vi "CreateArrayHeadersFromRoutineEntries.vi"(0 "Available Routines":string[][](table), 5 "error in":errorcluster) -> (14 "Available Routines out":string[][](table), 15 "Column Headers":string[](array[string]), 16 "Row Headers":string[](array[string]), 19 "error out":errorcluster)   [LabVIEW 2014]
doc: "This VI creates the array headers for the fast alignment routine managing VIs."
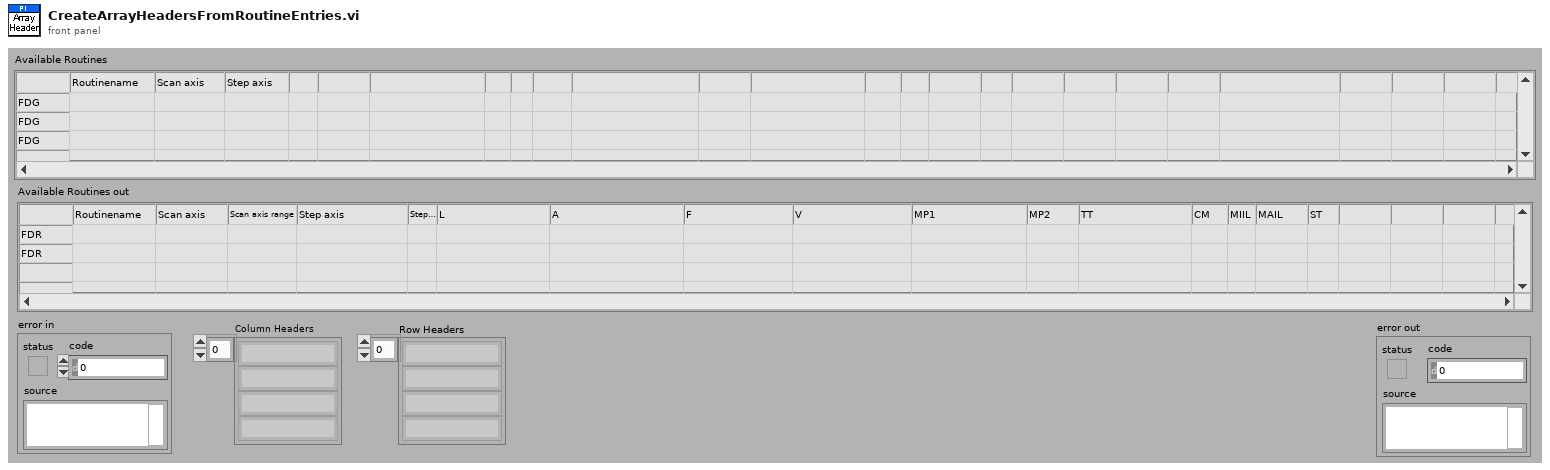
[diagram p1: front panel]
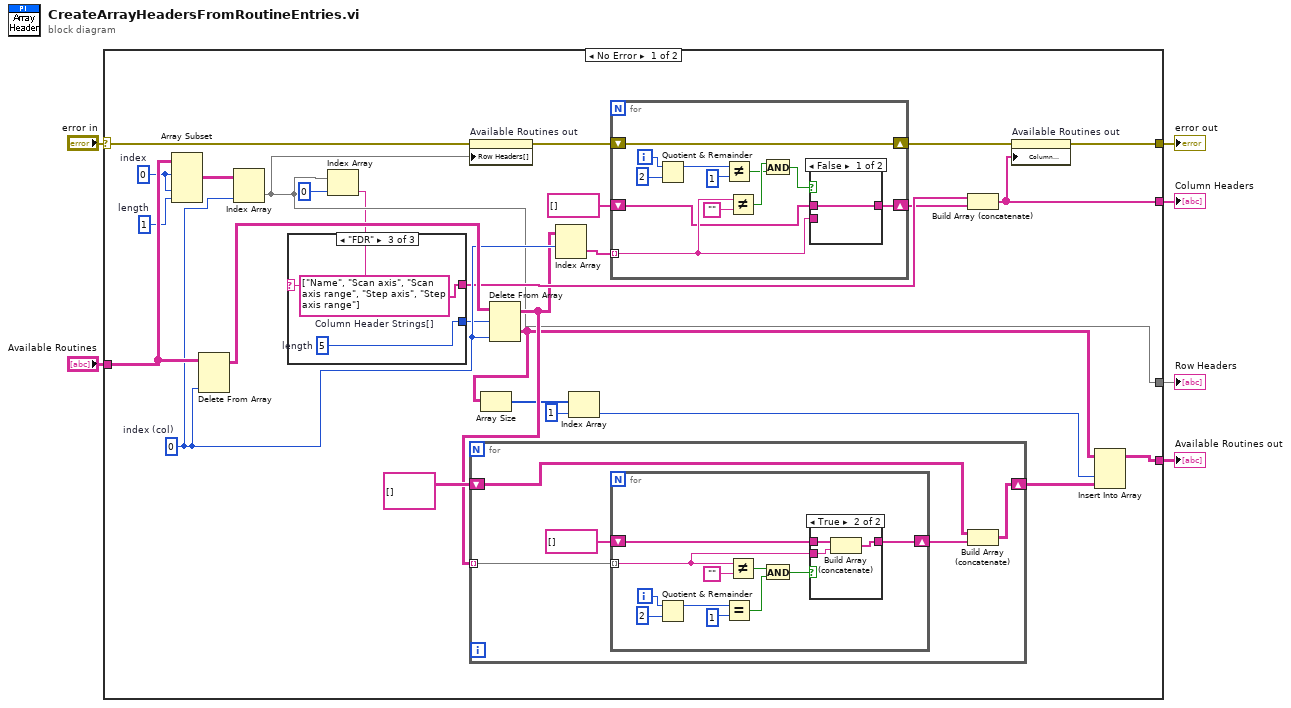
[diagram p0: block diagram]
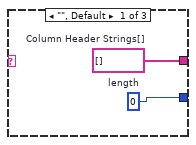
[diagram p2: hidden frame]
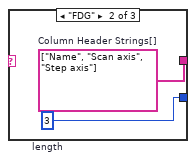
[diagram p3: hidden frame]
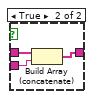
[diagram p5: hidden frame]
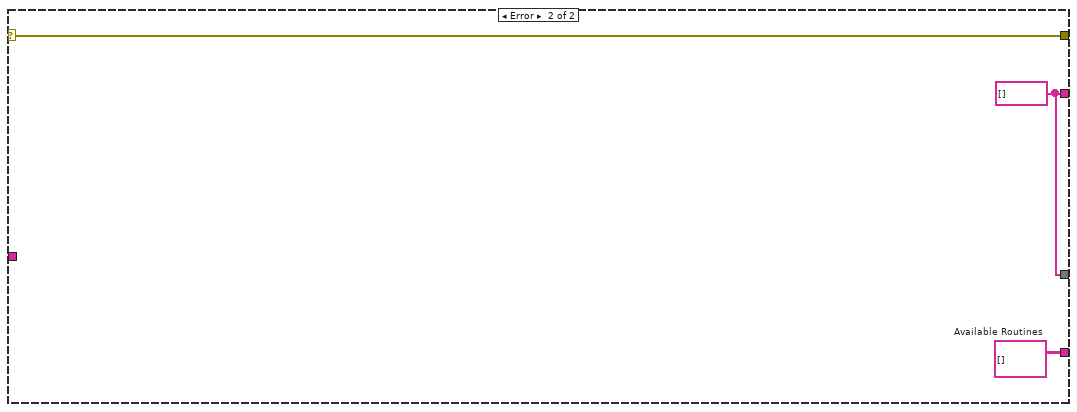
[diagram p6: hidden frame]
diagram:
  n1 = case shown="No Error" "error in" {
    selector: "error in" -> [w8 w78]
    tunnel: "Available Routines" -> [w33 _]
    tunnel: [w32 w77] -> w5
    tunnel: [w31 w78] -> w4
    tunnel: [w30 w76] -> w2
    tunnel: [w11 w76] -> w1
    frame No Error {
      w25 = 0  # index (col)
      w28 = 1  # length
      w29 = 0  # index
      n2 = Array Subset(array=w33, index (row)=w29, index (col)=w29, length (col)=w28) -> (w27:string[][])  [unwired: 1 in]
      n3 = Delete From Array(array=w33, index (col)=w25) -> (array with subset deleted=w26:string[][])  [unwired: 2 in, 1 out]
      n4 = Index Array(array=w27, index (col)=w25) -> (element=w11:string[])  [unwired: 1 in]
      n5 = Index Array(array=w11, index=0) -> (element=w9:string)
      n6 = case shown="\"FDR\"" w9 {
        tunnel: [w35 w37 w39] -> w22
        tunnel: [w34 w36 w38] -> w7
        frame "", Default {
          w34 = 0  # length
          w35 = string[] []  # Column Header Strings[]
        }
        frame "FDG" {
          w36 = 3  # length
          w37 = string[] ["Name", "Scan axis", "Step axis"]  # Column Header Strings[]
        }
        frame "FDR" {
          w38 = 5  # length
          w39 = string[] ["Name", "Scan axis", "Scan axis range", "Step axis", "Step axis range"]  # Column Header Strings[]
        }
      }
      n7 = property on="Available Routines out" class="Tbl (strict)"(error in=w8, "Row Headers[]"=w11) -> (error out=w23:errorcluster)  [unwired: 1 in, 1 out]
      n8 = Delete From Array(array=w26, length=w7, index (col)=w25) -> (deleted portion=w15:string[][], array with subset deleted=w17:string[][])  [unwired: 1 in]
      n9 = for {
        tunnel: w17 -> [w44] mode=indexing
        shift-right: [w41] -> w16
        shift-left: string[][] [] -> [w43]
        n10 = for {
          tunnel: w44 -> [w52] mode=indexing
          shift-right: [w50] -> w42
          shift-left: string[] [] -> [w51]
          i -> [w49]
          n11 = Quotient & Remainder(x=w49, y=2) -> (x-y*floor(x/y)=w47:i32)  [unwired: 1 out]
          n12 = Equal?(x=w47, y=1) -> (x = y?=w45:bool)
          n13 = Not Equal?(x=w52, y="") -> (x != y?=w54:bool)
          n14 = And(x=w54, y=w45) -> (x .and. y?=w53:bool)
          n15 = case shown="True" w53 {
            tunnel: w52 -> [_ w58]
            tunnel: w51 -> [w56 w59]
            tunnel: [w56 w57] -> w50
            frame False {
            }
            frame True {
              n16 = Build Array (concatenate)(w59, w58) -> (w57:string[])
            }
          }
        }
        n17 = Build Array (concatenate)(w43, w42) -> (w41:string[][])
      }
      n18 = Array Size(array=w15) -> (size(s)=w14:i32[])
      n19 = Index Array(array=w17, index (row)=w25) -> (element=w24:string[])  [unwired: 1 in]
      n20 = Index Array(array=w14, index=1) -> (element=w12:i32)
      n21 = for {
        tunnel: w24 -> [w68] mode=indexing
        shift-right: [w66] -> w21
        shift-left: string[] [] -> [w67]
        shift-right: [w60] -> w19
        shift-left: w23 -> [w60]
        i -> [w65]
        n22 = Quotient & Remainder(x=w65, y=2) -> (x-y*floor(x/y)=w63:i32)  [unwired: 1 out]
        n23 = Not Equal?(x=w63, y=1) -> (x != y?=w61:bool)
        n24 = Not Equal?(x=w68, y="") -> (x != y?=w70:bool)
        n25 = And(x=w70, y=w61) -> (x .and. y?=w69:bool)
        n26 = case shown="False" w69 {
          tunnel: w68 -> [_ w74]
          tunnel: w67 -> [w72 w75]
          tunnel: [w72 w73] -> w66
          frame False {
          }
          frame True {
            n27 = Build Array (concatenate)(w75, w74) -> (w73:string[])
          }
        }
      }
      n28 = Build Array (concatenate)(w22, w21) -> (w30:string[])
      n29 = property on="Available Routines out" class="Tbl (strict)"(error in=w19, "Column Headers[]"=w30) -> (error out=w31:errorcluster)  [unwired: 1 in, 1 out]
      n30 = Insert Into Array(array=w15, index (col)=w12, new element=w16) -> (w32:string[][])  [unwired: 1 in]
    }
    frame Error {
      w76 = string[] []
      w77 = string[][] []  # Available Routines
    }
  }
  "Available Routines out" <- w5
  "error out" <- w4
  "Column Headers" <- w2
  "Row Headers" <- w1
